vi "ProfilerTest.vi"() -> ()   [LabVIEW 2014] (continued)
{"Time"=28.20000000000161, "delVelocity"=0.0}, {"Time"=28.21000000000161, "delVelocity"=0.0}, {"Time"=28.220000000001612, "delVelocity"=0.0}, {"Time"=28.230000000001613, "delVelocity"=0.0}, {"Time"=28.240000000001615, "delVelocity"=0.0}, {"Time"=28.250000000001616, "delVelocity"=0.0}, {"Time"=28.260000000001618, "delVelocity"=0.0}, {"Time"=28.27000000000162, "delVelocity"=0.0}, {"Time"=28.28000000000162, "delVelocity"=0.0}, {"Time"=28.290000000001623, "delVelocity"=0.0}, {"Time"=28.300000000001624, "delVelocity"=0.0}, {"Time"=28.310000000001626, "delVelocity"=0.0}, {"Time"=28.320000000001627, "delVelocity"=0.0}, {"Time"=28.33000000000163, "delVelocity"=0.0}, {"Time"=28.34000000000163, "delVelocity"=0.0}, {"Time"=28.350000000001632, "delVelocity"=0.0}, {"Time"=28.360000000001634, "delVelocity"=0.0}, {"Time"=28.370000000001635, "delVelocity"=0.0}, {"Time"=28.380000000001637, "delVelocity"=0.0}, {"Time"=28.39000000000164, "delVelocity"=0.0}, {"Time"=28.40000000000164, "delVelocity"=0.0}, {"Time"=28.41000000000164, "delVelocity"=0.0}, {"Time"=28.420000000001643, "delVelocity"=0.0}, {"Time"=28.430000000001645, "delVelocity"=0.0}, {"Time"=28.440000000001646, "delVelocity"=0.0}, {"Time"=28.450000000001648, "delVelocity"=0.0}, {"Time"=28.46000000000165, "delVelocity"=0.0}, {"Time"=28.47000000000165, "delVelocity"=0.0}, {"Time"=28.480000000001652, "delVelocity"=0.0}, {"Time"=28.490000000001654, "delVelocity"=0.0}, {"Time"=28.500000000001656, "delVelocity"=0.0}, {"Time"=28.510000000001657, "delVelocity"=0.0}, {"Time"=28.52000000000166, "delVelocity"=0.0}, {"Time"=28.53000000000166, "delVelocity"=0.0}, {"Time"=28.540000000001662, "delVelocity"=0.0}, {"Time"=28.550000000001663, "delVelocity"=0.0}, {"Time"=28.560000000001665, "delVelocity"=0.0}, {"Time"=28.570000000001667, "delVelocity"=0.0}, {"Time"=28.580000000001668, "delVelocity"=0.0}, {"Time"=28.59000000000167, "delVelocity"=0.0}, {"Time"=28.60000000000167, "delVelocity"=0.0}, {"Time"=28.610000000001673, "delVelocity"=0.0}, {"Time"=28.620000000001674, "delVelocity"=0.0}, {"Time"=28.630000000001676, "delVelocity"=0.0}, {"Time"=28.640000000001677, "delVelocity"=0.0}, {"Time"=28.65000000000168, "delVelocity"=0.0}, {"Time"=28.66000000000168, "delVelocity"=0.0}, {"Time"=28.670000000001682, "delVelocity"=0.0}, {"Time"=28.680000000001684, "delVelocity"=0.0}, {"Time"=28.690000000001685, "delVelocity"=0.0}, {"Time"=28.700000000001687, "delVelocity"=0.0}, {"Time"=28.71000000000169, "delVelocity"=0.0}, {"Time"=28.72000000000169, "delVelocity"=0.0}, {"Time"=28.73000000000169, "delVelocity"=0.0}, {"Time"=28.740000000001693, "delVelocity"=0.0}, {"Time"=28.750000000001695, "delVelocity"=0.0}, {"Time"=28.760000000001696, "delVelocity"=0.0}, {"Time"=28.770000000001698, "delVelocity"=0.0}, {"Time"=28.7800000000017, "delVelocity"=0.0}, {"Time"=28.7900000000017, "delVelocity"=0.0}, {"Time"=28.800000000001702, "delVelocity"=0.0}, {"Time"=28.810000000001704, "delVelocity"=0.0}, {"Time"=28.820000000001706, "delVelocity"=0.0}, {"Time"=28.830000000001707, "delVelocity"=0.0}, {"Time"=28.84000000000171, "delVelocity"=0.0}, {"Time"=28.85000000000171, "delVelocity"=0.0}, {"Time"=28.860000000001712, "delVelocity"=0.0}, {"Time"=28.870000000001713, "delVelocity"=0.0}, {"Time"=28.880000000001715, "delVelocity"=0.0}, {"Time"=28.890000000001717, "delVelocity"=0.0}, {"Time"=28.900000000001718, "delVelocity"=0.0}, {"Time"=28.91000000000172, "delVelocity"=0.0}, {"Time"=28.92000000000172, "delVelocity"=0.0}, {"Time"=28.930000000001723, "delVelocity"=0.0}, {"Time"=28.940000000001724, "delVelocity"=0.0}, {"Time"=28.950000000001726, "delVelocity"=0.0}, {"Time"=28.960000000001727, "delVelocity"=0.0}, {"Time"=28.97000000000173, "delVelocity"=0.0}, {"Time"=28.98000000000173, "delVelocity"=0.0}, {"Time"=28.990000000001732, "delVelocity"=0.0}, {"Time"=29.000000000001734, "delVelocity"=0.0}, {"Time"=29.010000000001735, "delVelocity"=0.0}, {"Time"=29.020000000001737, "delVelocity"=0.0}, {"Time"=29.03000000000174, "delVelocity"=0.0}, {"Time"=29.04000000000174, "delVelocity"=0.0}, {"Time"=29.05000000000174, "delVelocity"=0.0}, {"Time"=29.060000000001743, "delVelocity"=0.0}, {"Time"=29.070000000001745, "delVelocity"=0.0}, {"Time"=29.080000000001746, "delVelocity"=0.0}, {"Time"=29.090000000001748, "delVelocity"=0.0}, {"Time"=29.10000000000175, "delVelocity"=0.0}, {"Time"=29.11000000000175, "delVelocity"=0.0}, {"Time"=29.120000000001752, "delVelocity"=0.0}, {"Time"=29.130000000001754, "delVelocity"=0.0}, {"Time"=29.140000000001756, "delVelocity"=0.0}, {"Time"=29.150000000001757, "delVelocity"=0.0}, {"Time"=29.16000000000176, "delVelocity"=0.0}, {"Time"=29.17000000000176, "delVelocity"=0.0}, {"Time"=29.180000000001762, "delVelocity"=0.0}, {"Time"=29.190000000001763, "delVelocity"=0.0}, {"Time"=29.200000000001765, "delVelocity"=0.0}, {"Time"=29.210000000001767, "delVelocity"=0.0}, {"Time"=29.220000000001768, "delVelocity"=0.0}, {"Time"=29.23000000000177, "delVelocity"=0.0}, {"Time"=29.24000000000177, "delVelocity"=0.0}, {"Time"=29.250000000001773, "delVelocity"=0.0}, {"Time"=29.260000000001774, "delVelocity"=0.0}, {"Time"=29.270000000001776, "delVelocity"=0.0}, {"Time"=29.280000000001777, "delVelocity"=0.0}, {"Time"=29.29000000000178, "delVelocity"=0.0}, {"Time"=29.30000000000178, "delVelocity"=0.0}, {"Time"=29.310000000001782, "delVelocity"=0.0}, {"Time"=29.320000000001784, "delVelocity"=0.0}, {"Time"=29.330000000001785, "delVelocity"=0.0}, {"Time"=29.340000000001787, "delVelocity"=0.0}, {"Time"=29.35000000000179, "delVelocity"=0.0}, {"Time"=29.36000000000179, "delVelocity"=0.0}, {"Time"=29.37000000000179, "delVelocity"=0.0}, {"Time"=29.380000000001793, "delVelocity"=0.0}, {"Time"=29.390000000001795, "delVelocity"=0.0}, {"Time"=29.400000000001796, "delVelocity"=0.0}, {"Time"=29.410000000001798, "delVelocity"=0.0}, {"Time"=29.4200000000018, "delVelocity"=0.0}, {"Time"=29.4300000000018, "delVelocity"=0.0}, {"Time"=29.440000000001803, "delVelocity"=0.0}, {"Time"=29.450000000001804, "delVelocity"=0.0}, {"Time"=29.460000000001806, "delVelocity"=0.0}, {"Time"=29.470000000001807, "delVelocity"=0.0}, {"Time"=29.48000000000181, "delVelocity"=0.0}, {"Time"=29.49000000000181, "delVelocity"=0.0}, {"Time"=29.500000000001812, "delVelocity"=0.0}, {"Time"=29.510000000001813, "delVelocity"=0.0}, {"Time"=29.520000000001815, "delVelocity"=0.0}, {"Time"=29.530000000001817, "delVelocity"=0.0}, {"Time"=29.540000000001818, "delVelocity"=0.0}, {"Time"=29.55000000000182, "delVelocity"=0.0}, {"Time"=29.56000000000182, "delVelocity"=0.0}, {"Time"=29.570000000001823, "delVelocity"=0.0}, {"Time"=29.580000000001824, "delVelocity"=0.0}, {"Time"=29.590000000001826, "delVelocity"=0.0}, {"Time"=29.600000000001828, "delVelocity"=0.0}, {"Time"=29.61000000000183, "delVelocity"=0.0}, {"Time"=29.62000000000183, "delVelocity"=0.0}, {"Time"=29.630000000001832, "delVelocity"=0.0}, {"Time"=29.640000000001834, "delVelocity"=0.0}, {"Time"=29.650000000001835, "delVelocity"=0.0}, {"Time"=29.660000000001837, "delVelocity"=0.0}, {"Time"=29.67000000000184, "delVelocity"=0.0}, {"Time"=29.68000000000184, "delVelocity"=0.0}, {"Time"=29.69000000000184, "delVelocity"=0.0}, {"Time"=29.700000000001843, "delVelocity"=0.0}, {"Time"=29.710000000001845, "delVelocity"=0.0}, {"Time"=29.720000000001846, "delVelocity"=0.0}, {"Time"=29.730000000001848, "delVelocity"=0.0}, {"Time"=29.74000000000185, "delVelocity"=0.0}, {"Time"=29.75000000000185, "delVelocity"=0.0}, {"Time"=29.760000000001853, "delVelocity"=0.0}, {"Time"=29.770000000001854, "delVelocity"=0.0}, {"Time"=29.780000000001856, "delVelocity"=0.0}, {"Time"=29.790000000001857, "delVelocity"=0.0}, {"Time"=29.80000000000186, "delVelocity"=0.0}, {"Time"=29.81000000000186, "delVelocity"=0.0}, {"Time"=29.820000000001862, "delVelocity"=0.0}, {"Time"=29.830000000001863, "delVelocity"=0.0}, {"Time"=29.840000000001865, "delVelocity"=0.0}, {"Time"=29.850000000001867, "delVelocity"=0.0}, {"Time"=29.860000000001868, "delVelocity"=0.0}, {"Time"=29.87000000000187, "delVelocity"=0.0}, {"Time"=29.88000000000187, "delVelocity"=0.0}, {"Time"=29.890000000001873, "delVelocity"=0.0}, {"Time"=29.900000000001874, "delVelocity"=0.0}, {"Time"=29.910000000001876, "delVelocity"=0.0}, {"Time"=29.920000000001878, "delVelocity"=0.0}, {"Time"=29.93000000000188, "delVelocity"=0.0}, {"Time"=29.94000000000188, "delVelocity"=0.0}, {"Time"=29.950000000001882, "delVelocity"=0.0}, {"Time"=29.960000000001884, "delVelocity"=0.0}, {"Time"=29.970000000001885, "delVelocity"=0.0}, {"Time"=29.980000000001887, "delVelocity"=0.0}, {"Time"=29.99000000000189, "delVelocity"=0.0}, {"Time"=30.00000000000189, "delVelocity"=0.0}, {"Time"=30.01000000000189, "delVelocity"=0.0}, {"Time"=30.020000000001893, "delVelocity"=0.0}, {"Time"=30.030000000001895, "delVelocity"=0.0}, {"Time"=30.040000000001896, "delVelocity"=0.0}, {"Time"=30.050000000001898, "delVelocity"=0.0}, {"Time"=30.0600000000019, "delVelocity"=0.0}, {"Time"=30.0700000000019, "delVelocity"=0.0}, {"Time"=30.080000000001903, "delVelocity"=0.0}, {"Time"=30.090000000001904, "delVelocity"=0.0}, {"Time"=30.100000000001906, "delVelocity"=0.0}, {"Time"=30.110000000001907, "delVelocity"=0.0}, {"Time"=30.12000000000191, "delVelocity"=0.0}, {"Time"=30.13000000000191, "delVelocity"=0.0}, {"Time"=30.140000000001912, "delVelocity"=0.0}, {"Time"=30.150000000001913, "delVelocity"=0.0}, {"Time"=30.160000000001915, "delVelocity"=0.0}, {"Time"=30.170000000001917, "delVelocity"=0.0}, {"Time"=30.180000000001918, "delVelocity"=0.0}, {"Time"=30.19000000000192, "delVelocity"=0.0}, {"Time"=30.20000000000192, "delVelocity"=0.0}, {"Time"=30.210000000001923, "delVelocity"=0.0}, {"Time"=30.220000000001924, "delVelocity"=0.0}, {"Time"=30.230000000001926, "delVelocity"=0.0}, {"Time"=30.240000000001928, "delVelocity"=0.0}, {"Time"=30.25000000000193, "delVelocity"=0.0}, {"Time"=30.26000000000193, "delVelocity"=0.0}, {"Time"=30.270000000001932, "delVelocity"=0.0}, {"Time"=30.280000000001934, "delVelocity"=0.0}, {"Time"=30.290000000001935, "delVelocity"=0.0}, {"Time"=30.300000000001937, "delVelocity"=0.0}, {"Time"=30.31000000000194, "delVelocity"=0.0}, {"Time"=30.32000000000194, "delVelocity"=0.0}, {"Time"=30.33000000000194, "delVelocity"=0.0}, {"Time"=30.340000000001943, "delVelocity"=0.0}, {"Time"=30.350000000001945, "delVelocity"=0.0}, {"Time"=30.360000000001946, "delVelocity"=0.0}, {"Time"=30.370000000001948, "delVelocity"=0.0}, {"Time"=30.38000000000195, "delVelocity"=0.0}, {"Time"=30.39000000000195, "delVelocity"=0.0}, {"Time"=30.400000000001953, "delVelocity"=0.0}, {"Time"=30.410000000001954, "delVelocity"=0.0}, {"Time"=30.420000000001956, "delVelocity"=0.0}, {"Time"=30.430000000001957, "delVelocity"=0.0}, {"Time"=30.44000000000196, "delVelocity"=0.0}, {"Time"=30.45000000000196, "delVelocity"=0.0}, {"Time"=30.460000000001962, "delVelocity"=0.0}, {"Time"=30.470000000001964, "delVelocity"=0.0}, {"Time"=30.480000000001965, "delVelocity"=0.0}, {"Time"=30.490000000001967, "delVelocity"=0.0}, {"Time"=30.500000000001968, "delVelocity"=0.0}, {"Time"=30.51000000000197, "delVelocity"=0.0}, {"Time"=30.52000000000197, "delVelocity"=0.0}, {"Time"=30.530000000001973, "delVelocity"=0.0}, {"Time"=30.540000000001974, "delVelocity"=0.0}, {"Time"=30.550000000001976, "delVelocity"=0.0}, {"Time"=30.560000000001978, "delVelocity"=0.0}, {"Time"=30.57000000000198, "delVelocity"=0.0}, {"Time"=30.58000000000198, "delVelocity"=0.0}, {"Time"=30.590000000001982, "delVelocity"=0.0}, {"Time"=30.600000000001984, "delVelocity"=0.0}, {"Time"=30.610000000001985, "delVelocity"=0.0}, {"Time"=30.620000000001987, "delVelocity"=0.0}, {"Time"=30.63000000000199, "delVelocity"=0.0}, {"Time"=30.64000000000199, "delVelocity"=0.0}, {"Time"=30.65000000000199, "delVelocity"=0.0}, {"Time"=30.660000000001993, "delVelocity"=0.0}, {"Time"=30.670000000001995, "delVelocity"=0.0}, {"Time"=30.680000000001996, "delVelocity"=0.0}, {"Time"=30.690000000001998, "delVelocity"=0.0}, {"Time"=30.700000000002, "delVelocity"=0.0}, {"Time"=30.710000000002, "delVelocity"=0.0}, {"Time"=30.720000000002003, "delVelocity"=0.0}, {"Time"=30.730000000002004, "delVelocity"=0.0}, {"Time"=30.740000000002006, "delVelocity"=0.0}, {"Time"=30.750000000002007, "delVelocity"=0.0}, {"Time"=30.76000000000201, "delVelocity"=0.0}, {"Time"=30.77000000000201, "delVelocity"=0.0}, {"Time"=30.780000000002012, "delVelocity"=0.0}, {"Time"=30.790000000002014, "delVelocity"=0.0}, {"Time"=30.800000000002015, "delVelocity"=0.0}, {"Time"=30.810000000002017, "delVelocity"=0.0}, {"Time"=30.82000000000202, "delVelocity"=0.0}, {"Time"=30.83000000000202, "delVelocity"=0.0}, {"Time"=30.84000000000202, "delVelocity"=0.0}, {"Time"=30.850000000002023, "delVelocity"=0.0}, {"Time"=30.860000000002024, "delVelocity"=0.0}, {"Time"=30.870000000002026, "delVelocity"=0.0}, {"Time"=30.880000000002028, "delVelocity"=0.0}, {"Time"=30.89000000000203, "delVelocity"=0.0}, {"Time"=30.90000000000203, "delVelocity"=0.0}, {"Time"=30.910000000002032, "delVelocity"=0.0}, {"Time"=30.920000000002034, "delVelocity"=0.0}, {"Time"=30.930000000002035, "delVelocity"=0.0}, {"Time"=30.940000000002037, "delVelocity"=0.0}, {"Time"=30.95000000000204, "delVelocity"=0.0}, {"Time"=30.96000000000204, "delVelocity"=0.0}, {"Time"=30.97000000000204, "delVelocity"=0.0}, {"Time"=30.980000000002043, "delVelocity"=0.0}, {"Time"=30.990000000002045, "delVelocity"=0.0}, {"Time"=31.000000000002046, "delVelocity"=0.0}, {"Time"=31.010000000002048, "delVelocity"=0.0}, {"Time"=31.02000000000205, "delVelocity"=0.0}, {"Time"=31.03000000000205, "delVelocity"=0.0}, {"Time"=31.040000000002053, "delVelocity"=0.0}, {"Time"=31.050000000002054, "delVelocity"=0.0}, {"Time"=31.060000000002056, "delVelocity"=0.0}, {"Time"=31.070000000002057, "delVelocity"=0.0}, {"Time"=31.08000000000206, "delVelocity"=0.0}, {"Time"=31.09000000000206, "delVelocity"=0.0}, {"Time"=31.100000000002062, "delVelocity"=0.0}, {"Time"=31.110000000002064, "delVelocity"=0.0}, {"Time"=31.120000000002065, "delVelocity"=0.0}, {"Time"=31.130000000002067, "delVelocity"=0.0}, {"Time"=31.14000000000207, "delVelocity"=0.0}, {"Time"=31.15000000000207, "delVelocity"=0.0}, {"Time"=31.16000000000207, "delVelocity"=0.0}, {"Time"=31.170000000002073, "delVelocity"=0.0}, {"Time"=31.180000000002075, "delVelocity"=0.0}, {"Time"=31.190000000002076, "delVelocity"=0.0}, {"Time"=31.200000000002078, "delVelocity"=0.0}, {"Time"=31.21000000000208, "delVelocity"=0.0}, {"Time"=31.22000000000208, "delVelocity"=0.0}, {"Time"=31.230000000002082, "delVelocity"=0.0}, {"Time"=31.240000000002084, "delVelocity"=0.0}, {"Time"=31.250000000002085, "delVelocity"=0.0}, {"Time"=31.260000000002087, "delVelocity"=0.0}, {"Time"=31.27000000000209, "delVelocity"=0.0}, {"Time"=31.28000000000209, "delVelocity"=0.0}, {"Time"=31.29000000000209, "delVelocity"=0.0}, {"Time"=31.300000000002093, "delVelocity"=0.0}, {"Time"=31.310000000002095, "delVelocity"=0.0}, {"Time"=31.320000000002096, "delVelocity"=0.0}, {"Time"=31.330000000002098, "delVelocity"=0.0}, {"Time"=31.3400000000021, "delVelocity"=0.0}, {"Time"=31.3500000000021, "delVelocity"=0.0}, {"Time"=31.360000000002103, "delVelocity"=0.0}, {"Time"=31.370000000002104, "delVelocity"=0.0}, {"Time"=31.380000000002106, "delVelocity"=0.0}, {"Time"=31.390000000002107, "delVelocity"=0.0}, {"Time"=31.40000000000211, "delVelocity"=0.0}, {"Time"=31.41000000000211, "delVelocity"=0.0}, {"Time"=31.420000000002112, "delVelocity"=0.0}, {"Time"=31.430000000002114, "delVelocity"=0.0}, {"Time"=31.440000000002115, "delVelocity"=0.0}, {"Time"=31.450000000002117, "delVelocity"=0.0}, {"Time"=31.46000000000212, "delVelocity"=0.0}, {"Time"=31.47000000000212, "delVelocity"=0.0}, {"Time"=31.48000000000212, "delVelocity"=0.0}, {"Time"=31.490000000002123, "delVelocity"=0.0}, {"Time"=31.500000000002125, "delVelocity"=0.0}, {"Time"=31.510000000002126, "delVelocity"=0.0}, {"Time"=31.520000000002128, "delVelocity"=0.0}, {"Time"=31.53000000000213, "delVelocity"=0.0}, {"Time"=31.54000000000213, "delVelocity"=0.0}, {"Time"=31.550000000002132, "delVelocity"=0.0}, {"Time"=31.560000000002134, "delVelocity"=0.0}, {"Time"=31.570000000002135, "delVelocity"=0.0}, {"Time"=31.580000000002137, "delVelocity"=0.0}, {"Time"=31.59000000000214, "delVelocity"=0.0}, {"Time"=31.60000000000214, "delVelocity"=0.0}, {"Time"=31.61000000000214, "delVelocity"=0.0}, {"Time"=31.620000000002143, "delVelocity"=0.0}, {"Time"=31.630000000002145, "delVelocity"=0.0}, {"Time"=31.640000000002146, "delVelocity"=0.0}, {"Time"=31.650000000002148, "delVelocity"=0.0}, {"Time"=31.66000000000215, "delVelocity"=0.0}, {"Time"=31.67000000000215, "delVelocity"=0.0}, {"Time"=31.680000000002153, "delVelocity"=0.0}, {"Time"=31.690000000002154, "delVelocity"=0.0}, {"Time"=31.700000000002156, "delVelocity"=0.0}, {"Time"=31.710000000002157, "delVelocity"=0.0}, {"Time"=31.72000000000216, "delVelocity"=0.0}, {"Time"=31.73000000000216, "delVelocity"=0.0}, {"Time"=31.740000000002162, "delVelocity"=0.0}, {"Time"=31.750000000002164, "delVelocity"=0.0}, {"Time"=31.760000000002165, "delVelocity"=0.0}, {"Time"=31.770000000002167, "delVelocity"=0.0}, {"Time"=31.78000000000217, "delVelocity"=0.0}, {"Time"=31.79000000000217, "delVelocity"=0.0}, {"Time"=31.80000000000217, "delVelocity"=0.0}, {"Time"=31.810000000002173, "delVelocity"=0.0}, {"Time"=31.820000000002175, "delVelocity"=0.0}, {"Time"=31.830000000002176, "delVelocity"=0.0}, {"Time"=31.840000000002178, "delVelocity"=0.0}, {"Time"=31.85000000000218, "delVelocity"=0.0}, {"Time"=31.86000000000218, "delVelocity"=0.0}, {"Time"=31.870000000002182, "delVelocity"=0.0}, {"Time"=31.880000000002184, "delVelocity"=0.0}, {"Time"=31.890000000002185, "delVelocity"=0.0}, {"Time"=31.900000000002187, "delVelocity"=0.0}, {"Time"=31.91000000000219, "delVelocity"=0.0}, {"Time"=31.92000000000219, "delVelocity"=0.0}, {"Time"=31.93000000000219, "delVelocity"=0.0}, {"Time"=31.940000000002193, "delVelocity"=0.0}, {"Time"=31.950000000002195, "delVelocity"=0.0}, {"Time"=31.960000000002196, "delVelocity"=0.0}, {"Time"=31.970000000002198, "delVelocity"=0.0}, {"Time"=31.9800000000022, "delVelocity"=0.0}, {"Time"=31.9900000000022, "delVelocity"=0.0}, {"Time"=32.0000000000022, "delVelocity"=0.0}, {"Time"=32.0100000000022, "delVelocity"=0.0}, {"Time"=32.0200000000022, "delVelocity"=0.0}, {"Time"=32.0300000000022, "delVelocity"=0.0}, {"Time"=32.040000000002195, "delVelocity"=0.0}, {"Time"=32.05000000000219, "delVelocity"=0.0}, {"Time"=32.06000000000219, "delVelocity"=0.0}, {"Time"=32.07000000000219, "delVelocity"=0.0}, {"Time"=32.08000000000219, "delVelocity"=0.0}, {"Time"=32.090000000002185, "delVelocity"=0.0}, {"Time"=32.10000000000218, "delVelocity"=0.0}, {"Time"=32.11000000000218, "delVelocity"=0.0}, {"Time"=32.12000000000218, "delVelocity"=0.0}, {"Time"=32.13000000000218, "delVelocity"=0.0}, {"Time"=32.140000000002175, "delVelocity"=0.0}, {"Time"=32.15000000000217, "delVelocity"=0.0}, {"Time"=32.16000000000217, "delVelocity"=0.0}, {"Time"=32.17000000000217, "delVelocity"=0.0}, {"Time"=32.18000000000217, "delVelocity"=0.0}, {"Time"=32.190000000002165, "delVelocity"=0.0}, {"Time"=32.20000000000216, "delVelocity"=0.0}, {"Time"=32.21000000000216, "delVelocity"=0.0}, {"Time"=32.22000000000216, "delVelocity"=0.0}, {"Time"=32.23000000000216, "delVelocity"=0.0}, {"Time"=32.240000000002155, "delVelocity"=0.0}, {"Time"=32.25000000000215, "delVelocity"=0.0}, {"Time"=32.26000000000215, "delVelocity"=0.0}, {"Time"=32.27000000000215, "delVelocity"=0.0}, {"Time"=32.28000000000215, "delVelocity"=0.0}, {"Time"=32.290000000002145, "delVelocity"=0.0}, {"Time"=32.30000000000214, "delVelocity"=0.0}, {"Time"=32.31000000000214, "delVelocity"=0.0}, {"Time"=32.32000000000214, "delVelocity"=0.0}, {"Time"=32.33000000000214, "delVelocity"=0.0}, {"Time"=32.340000000002135, "delVelocity"=0.0}, {"Time"=32.35000000000213, "delVelocity"=0.0}, {"Time"=32.36000000000213, "delVelocity"=0.0}, {"Time"=32.37000000000213, "delVelocity"=0.0}, {"Time"=32.38000000000213, "delVelocity"=0.0}, {"Time"=32.390000000002125, "delVelocity"=0.0}, {"Time"=32.40000000000212, "delVelocity"=0.0}, {"Time"=32.41000000000212, "delVelocity"=0.0}, {"Time"=32.42000000000212, "delVelocity"=0.0}, {"Time"=32.43000000000212, "delVelocity"=0.0}, {"Time"=32.440000000002115, "delVelocity"=0.0}, {"Time"=32.45000000000211, "delVelocity"=0.0}, {"Time"=32.46000000000211, "delVelocity"=0.0}, {"Time"=32.47000000000211, "delVelocity"=0.0}, {"Time"=32.48000000000211, "delVelocity"=0.0}, {"Time"=32.490000000002105, "delVelocity"=0.0}, {"Time"=32.5000000000021, "delVelocity"=0.0}, {"Time"=32.5100000000021, "delVelocity"=0.0}, {"Time"=32.5200000000021, "delVelocity"=0.0}, {"Time"=32.5300000000021, "delVelocity"=0.0}, {"Time"=32.540000000002095, "delVelocity"=0.0}, {"Time"=32.55000000000209, "delVelocity"=0.0}, {"Time"=32.56000000000209, "delVelocity"=0.0}, {"Time"=32.57000000000209, "delVelocity"=0.0}, {"Time"=32.58000000000209, "delVelocity"=0.0}, {"Time"=32.590000000002085, "delVelocity"=0.0}, {"Time"=32.60000000000208, "delVelocity"=0.0}, {"Time"=32.61000000000208, "delVelocity"=0.0}, {"Time"=32.62000000000208, "delVelocity"=0.0}, {"Time"=32.63000000000208, "delVelocity"=0.0}, {"Time"=32.640000000002075, "delVelocity"=0.0}, {"Time"=32.65000000000207, "delVelocity"=0.0}, {"Time"=32.66000000000207, "delVelocity"=0.0}, {"Time"=32.67000000000207, "delVelocity"=0.0}, {"Time"=32.68000000000207, "delVelocity"=0.0}, {"Time"=32.690000000002065, "delVelocity"=0.0}, {"Time"=32.70000000000206, "delVelocity"=0.0}, {"Time"=32.71000000000206, "delVelocity"=0.0}, {"Time"=32.72000000000206, "delVelocity"=0.0}, {"Time"=32.73000000000206, "delVelocity"=0.0}, {"Time"=32.740000000002055, "delVelocity"=0.0}, {"Time"=32.75000000000205, "delVelocity"=0.0}, {"Time"=32.76000000000205, "delVelocity"=0.0}, {"Time"=32.77000000000205, "delVelocity"=0.0}, {"Time"=32.78000000000205, "delVelocity"=0.0}, {"Time"=32.790000000002046, "delVelocity"=0.0}, {"Time"=32.80000000000204, "delVelocity"=0.0}, {"Time"=32.81000000000204, "delVelocity"=0.0}, {"Time"=32.82000000000204, "delVelocity"=0.0}, {"Time"=32.83000000000204, "delVelocity"=0.0}, {"Time"=32.840000000002036, "delVelocity"=0.0}, {"Time"=32.850000000002034, "delVelocity"=0.0}, {"Time"=32.86000000000203, "delVelocity"=0.0}, {"Time"=32.87000000000203, "delVelocity"=0.0}, {"Time"=32.88000000000203, "delVelocity"=0.0}, {"Time"=32.890000000002026, "delVelocity"=0.0}, {"Time"=32.900000000002024, "delVelocity"=0.0}, {"Time"=32.91000000000202, "delVelocity"=0.0}, {"Time"=32.92000000000202, "delVelocity"=0.0}, {"Time"=32.93000000000202, "delVelocity"=0.0}, {"Time"=32.940000000002016, "delVelocity"=0.0}, {"Time"=32.950000000002014, "delVelocity"=0.0}, {"Time"=32.96000000000201, "delVelocity"=0.0}, {"Time"=32.97000000000201, "delVelocity"=0.0}, {"Time"=32.98000000000201, "delVelocity"=0.0}, {"Time"=32.990000000002006, "delVelocity"=0.0}, {"Time"=33.000000000002004, "delVelocity"=0.0}, {"Time"=33.010000000002, "delVelocity"=0.0}, {"Time"=33.020000000002, "delVelocity"=0.0}, {"Time"=33.030000000002, "delVelocity"=0.0}, {"Time"=33.040000000001996, "delVelocity"=0.0}, {"Time"=33.050000000001994, "delVelocity"=0.0}, {"Time"=33.06000000000199, "delVelocity"=0.0}, {"Time"=33.07000000000199, "delVelocity"=0.0}, {"Time"=33.08000000000199, "delVelocity"=0.0}, {"Time"=33.090000000001986, "delVelocity"=0.0}, {"Time"=33.100000000001984, "delVelocity"=0.0}, {"Time"=33.11000000000198, "delVelocity"=0.0}, {"Time"=33.12000000000198, "delVelocity"=0.0}, {"Time"=33.13000000000198, "delVelocity"=0.0}, {"Time"=33.140000000001976, "delVelocity"=0.0}, {"Time"=33.150000000001974, "delVelocity"=0.0}, {"Time"=33.16000000000197, "delVelocity"=0.0}, {"Time"=33.17000000000197, "delVelocity"=0.0}, {"Time"=33.18000000000197, "delVelocity"=0.0}, {"Time"=33.190000000001966, "delVelocity"=0.0}, {"Time"=33.200000000001964, "delVelocity"=0.0}, {"Time"=33.21000000000196, "delVelocity"=0.0}, {"Time"=33.22000000000196, "delVelocity"=0.0}, {"Time"=33.23000000000196, "delVelocity"=0.0}, {"Time"=33.240000000001956, "delVelocity"=0.0}, {"Time"=33.250000000001954, "delVelocity"=0.0}, {"Time"=33.26000000000195, "delVelocity"=0.0}, {"Time"=33.27000000000195, "delVelocity"=0.0}, {"Time"=33.28000000000195, "delVelocity"=0.0}, {"Time"=33.290000000001946, "delVelocity"=0.0}, {"Time"=33.300000000001944, "delVelocity"=0.0}, {"Time"=33.31000000000194, "delVelocity"=0.0}, {"Time"=33.32000000000194, "delVelocity"=0.0}, {"Time"=33.33000000000194, "delVelocity"=0.0}, {"Time"=33.340000000001936, "delVelocity"=0.0}, {"Time"=33.350000000001934, "delVelocity"=0.0}, {"Time"=33.36000000000193, "delVelocity"=0.0}, {"Time"=33.37000000000193, "delVelocity"=0.0}, {"Time"=33.38000000000193, "delVelocity"=0.0}, {"Time"=33.390000000001926, "delVelocity"=0.0}, {"Time"=33.400000000001924, "delVelocity"=0.0}, {"Time"=33.41000000000192, "delVelocity"=0.0}, {"Time"=33.42000000000192, "delVelocity"=0.0}, {"Time"=33.43000000000192, "delVelocity"=0.0}, {"Time"=33.440000000001916, "delVelocity"=0.0}, {"Time"=33.450000000001914, "delVelocity"=0.0}, {"Time"=33.46000000000191, "delVelocity"=0.0}, {"Time"=33.47000000000191, "delVelocity"=0.0}, {"Time"=33.48000000000191, "delVelocity"=0.0}, {"Time"=33.490000000001906, "delVelocity"=0.0}, {"Time"=33.500000000001904, "delVelocity"=0.0}, {"Time"=33.5100000000019, "delVelocity"=0.0}, {"Time"=33.5200000000019, "delVelocity"=0.0}, {"Time"=33.5300000000019, "delVelocity"=0.0}, {"Time"=33.540000000001896, "delVelocity"=0.0}, {"Time"=33.550000000001894, "delVelocity"=0.0}, {"Time"=33.56000000000189, "delVelocity"=0.0}, {"Time"=33.57000000000189, "delVelocity"=0.0}, {"Time"=33.58000000000189, "delVelocity"=0.0}, {"Time"=33.590000000001886, "delVelocity"=0.0}, {"Time"=33.600000000001884, "delVelocity"=0.0}, {"Time"=33.61000000000188, "delVelocity"=0.0}, {"Time"=33.62000000000188, "delVelocity"=0.0}, {"Time"=33.63000000000188, "delVelocity"=0.0}, {"Time"=33.640000000001876, "delVelocity"=0.0}, {"Time"=33.650000000001874, "delVelocity"=0.0}, {"Time"=33.66000000000187, "delVelocity"=0.0}, {"Time"=33.67000000000187, "delVelocity"=0.0}, {"Time"=33.68000000000187, "delVelocity"=0.0}, {"Time"=33.69000000000187, "delVelocity"=0.0}, {"Time"=33.700000000001864, "delVelocity"=0.0}, {"Time"=33.71000000000186, "delVelocity"=0.0}, {"Time"=33.72000000000186, "delVelocity"=0.0}, {"Time"=33.73000000000186, "delVelocity"=0.0}, {"Time"=33.74000000000186, "delVelocity"=0.0}, {"Time"=33.750000000001855, "delVelocity"=0.0}, {"Time"=33.76000000000185, "delVelocity"=0.0}, {"Time"=33.77000000000185, "delVelocity"=0.0}, {"Time"=33.78000000000185, "delVelocity"=0.0}, {"Time"=33.79000000000185, "delVelocity"=0.0}, {"Time"=33.800000000001845, "delVelocity"=0.0}, {"Time"=33.81000000000184, "delVelocity"=0.0}, {"Time"=33.82000000000184, "delVelocity"=0.0}, {"Time"=33.83000000000184, "delVelocity"=0.0}, {"Time"=33.84000000000184, "delVelocity"=0.0}, {"Time"=33.850000000001835, "delVelocity"=0.0}, {"Time"=33.86000000000183, "delVelocity"=0.0}, {"Time"=33.87000000000183, "delVelocity"=0.0}, {"Time"=33.88000000000183, "delVelocity"=0.0}, {"Time"=33.89000000000183, "delVelocity"=0.0}, {"Time"=33.900000000001825, "delVelocity"=0.0}, {"Time"=33.91000000000182, "delVelocity"=0.0}, {"Time"=33.92000000000182, "delVelocity"=0.0}, {"Time"=33.93000000000182, "delVelocity"=0.0}, {"Time"=33.94000000000182, "delVelocity"=0.0}, {"Time"=33.950000000001815, "delVelocity"=0.0}, {"Time"=33.96000000000181, "delVelocity"=0.0}, {"Time"=33.97000000000181, "delVelocity"=0.0}, {"Time"=33.98000000000181, "delVelocity"=0.0}, {"Time"=33.99000000000181, "delVelocity"=0.0}, {"Time"=34.000000000001805, "delVelocity"=0.0}, {"Time"=34.0100000000018, "delVelocity"=0.0}, {"Time"=34.0200000000018, "delVelocity"=0.0}, {"Time"=34.0300000000018, "delVelocity"=0.0}, {"Time"=34.0400000000018, "delVelocity"=0.0}, {"Time"=34.050000000001795, "delVelocity"=0.0}, {"Time"=34.06000000000179, "delVelocity"=0.0}, {"Time"=34.07000000000179, "delVelocity"=0.0}, {"Time"=34.08000000000179, "delVelocity"=0.0}, {"Time"=34.09000000000179, "delVelocity"=0.0}, {"Time"=34.100000000001785, "delVelocity"=0.0}, {"Time"=34.11000000000178, "delVelocity"=0.0}, {"Time"=34.12000000000178, "delVelocity"=0.0}, {"Time"=34.13000000000178, "delVelocity"=0.0}, {"Time"=34.14000000000178, "delVelocity"=0.0}, {"Time"=34.150000000001775, "delVelocity"=0.0}, {"Time"=34.16000000000177, "delVelocity"=0.0}, {"Time"=34.17000000000177, "delVelocity"=0.0}, {"Time"=34.18000000000177, "delVelocity"=0.0}, {"Time"=34.19000000000177, "delVelocity"=0.0}, {"Time"=34.200000000001765, "delVelocity"=0.0}, {"Time"=34.21000000000176, "delVelocity"=0.0}, {"Time"=34.22000000000176, "delVelocity"=0.0}, {"Time"=34.23000000000176, "delVelocity"=0.0}, {"Time"=34.24000000000176, "delVelocity"=0.0}, {"Time"=34.250000000001755, "delVelocity"=0.0}, {"Time"=34.26000000000175, "delVelocity"=0.0}, {"Time"=34.27000000000175, "delVelocity"=0.0}, {"Time"=34.28000000000175, "delVelocity"=0.0}, {"Time"=34.29000000000175, "delVelocity"=0.0}, {"Time"=34.300000000001745, "delVelocity"=0.0}, {"Time"=34.31000000000174, "delVelocity"=0.0}, {"Time"=34.32000000000174, "delVelocity"=0.0}, {"Time"=34.33000000000174, "delVelocity"=0.0}, {"Time"=34.34000000000174, "delVelocity"=0.0}, {"Time"=34.350000000001735, "delVelocity"=0.0}, {"Time"=34.36000000000173, "delVelocity"=0.0}, {"Time"=34.37000000000173, "delVelocity"=0.0}, {"Time"=34.38000000000173, "delVelocity"=0.0}, {"Time"=34.39000000000173, "delVelocity"=0.0}, {"Time"=34.400000000001725, "delVelocity"=0.0}, {"Time"=34.41000000000172, "delVelocity"=0.0}, {"Time"=34.42000000000172, "delVelocity"=0.0}, {"Time"=34.43000000000172, "delVelocity"=0.0}, {"Time"=34.44000000000172, "delVelocity"=0.0}, {"Time"=34.450000000001715, "delVelocity"=0.0}, {"Time"=34.46000000000171, "delVelocity"=0.0}, {"Time"=34.47000000000171, "delVelocity"=0.0}, {"Time"=34.48000000000171, "delVelocity"=0.0}, {"Time"=34.49000000000171, "delVelocity"=0.0}, {"Time"=34.500000000001705, "delVelocity"=0.0}, {"Time"=34.5100000000017, "delVelocity"=0.0}, {"Time"=34.5200000000017, "delVelocity"=0.0}, {"Time"=34.5300000000017, "delVelocity"=0.0}, {"Time"=34.5400000000017, "delVelocity"=0.0}, {"Time"=34.550000000001695, "delVelocity"=0.0}, {"Time"=34.56000000000169, "delVelocity"=0.0}, {"Time"=34.57000000000169, "delVelocity"=0.0}, {"Time"=34.58000000000169, "delVelocity"=0.0}, {"Time"=34.59000000000169, "delVelocity"=0.0}, {"Time"=34.600000000001685, "delVelocity"=0.0}, {"Time"=34.61000000000168, "delVelocity"=0.0}, {"Time"=34.62000000000168, "delVelocity"=0.0}, {"Time"=34.63000000000168, "delVelocity"=0.0}, {"Time"=34.64000000000168, "delVelocity"=0.0}, {"Time"=34.650000000001675, "delVelocity"=0.0}, {"Time"=34.66000000000167, "delVelocity"=0.0}, {"Time"=34.67000000000167, "delVelocity"=0.0}, {"Time"=34.68000000000167, "delVelocity"=0.0}, {"Time"=34.69000000000167, "delVelocity"=0.0}, {"Time"=34.700000000001666, "delVelocity"=0.0}, {"Time"=34.71000000000166, "delVelocity"=0.0}, {"Time"=34.72000000000166, "delVelocity"=0.0}, {"Time"=34.73000000000166, "delVelocity"=0.0}, {"Time"=34.74000000000166, "delVelocity"=0.0}, {"Time"=34.750000000001656, "delVelocity"=0.0}, {"Time"=34.760000000001654, "delVelocity"=0.0}, {"Time"=34.77000000000165, "delVelocity"=0.0}, {"Time"=34.78000000000165, "delVelocity"=0.0}, {"Time"=34.79000000000165, "delVelocity"=0.0}, {"Time"=34.800000000001646, "delVelocity"=0.0}, {"Time"=34.810000000001644, "delVelocity"=0.0}, {"Time"=34.82000000000164, "delVelocity"=0.0}, {"Time"=34.83000000000164, "delVelocity"=0.0}, {"Time"=34.84000000000164, "delVelocity"=0.0}, {"Time"=34.850000000001636, "delVelocity"=0.0}, {"Time"=34.860000000001634, "delVelocity"=0.0}, {"Time"=34.87000000000163, "delVelocity"=0.0}, {"Time"=34.88000000000163, "delVelocity"=0.0}, {"Time"=34.89000000000163, "delVelocity"=0.0}, {"Time"=34.900000000001626, "delVelocity"=0.0}, {"Time"=34.910000000001624, "delVelocity"=0.0}, {"Time"=34.92000000000162, "delVelocity"=0.0}, {"Time"=34.93000000000162, "delVelocity"=0.0}, {"Time"=34.94000000000162, "delVelocity"=0.0}, {"Time"=34.950000000001616, "delVelocity"=0.0}, {"Time"=34.960000000001614, "delVelocity"=0.0}, {"Time"=34.97000000000161, "delVelocity"=0.0}, {"Time"=34.98000000000161, "delVelocity"=0.0}, {"Time"=34.99000000000161, "delVelocity"=0.0}, {"Time"=35.000000000001606, "delVelocity"=0.0}, {"Time"=35.010000000001604, "delVelocity"=0.0}, {"Time"=35.0200000000016, "delVelocity"=0.0}, {"Time"=35.0300000000016, "delVelocity"=0.0}, {"Time"=35.0400000000016, "delVelocity"=0.0}, {"Time"=35.050000000001596, "delVelocity"=0.0}, {"Time"=35.060000000001594, "delVelocity"=0.0}, {"Time"=35.07000000000159, "delVelocity"=0.0}, {"Time"=35.08000000000159, "delVelocity"=0.0}, {"Time"=35.09000000000159, "delVelocity"=0.0}, {"Time"=35.100000000001586, "delVelocity"=0.0}, {"Time"=35.110000000001584, "delVelocity"=0.0}, {"Time"=35.12000000000158, "delVelocity"=0.0}, {"Time"=35.13000000000158, "delVelocity"=0.0}, {"Time"=35.14000000000158, "delVelocity"=0.0}, {"Time"=35.150000000001576, "delVelocity"=0.0}, {"Time"=35.160000000001574, "delVelocity"=0.0}, {"Time"=35.17000000000157, "delVelocity"=0.0}, {"Time"=35.18000000000157, "delVelocity"=0.0}, {"Time"=35.19000000000157, "delVelocity"=0.0}, {"Time"=35.200000000001566, "delVelocity"=0.0}, {"Time"=35.210000000001564, "delVelocity"=0.0}, {"Time"=35.22000000000156, "delVelocity"=0.0}, {"Time"=35.23000000000156, "delVelocity"=0.0}, {"Time"=35.24000000000156, "delVelocity"=0.0}, {"Time"=35.250000000001556, "delVelocity"=0.0}, {"Time"=35.260000000001554, "delVelocity"=0.0}, {"Time"=35.27000000000155, "delVelocity"=0.0}, {"Time"=35.28000000000155, "delVelocity"=0.0}, {"Time"=35.29000000000155, "delVelocity"=0.0}, {"Time"=35.300000000001546, "delVelocity"=0.0}, {"Time"=35.310000000001544, "delVelocity"=0.0}, {"Time"=35.32000000000154, "delVelocity"=0.0}, {"Time"=35.33000000000154, "delVelocity"=0.0}, {"Time"=35.34000000000154, "delVelocity"=0.0}, {"Time"=35.350000000001536, "delVelocity"=0.0}, {"Time"=35.360000000001534, "delVelocity"=0.0}, {"Time"=35.37000000000153, "delVelocity"=0.0}, {"Time"=35.38000000000153, "delVelocity"=0.0}, {"Time"=35.39000000000153, "delVelocity"=0.0}, {"Time"=35.400000000001526, "delVelocity"=0.0}, {"Time"=35.410000000001524, "delVelocity"=0.0}, {"Time"=35.42000000000152, "delVelocity"=0.0}, {"Time"=35.43000000000152, "delVelocity"=0.0}, {"Time"=35.44000000000152, "delVelocity"=0.0}, {"Time"=35.450000000001516, "delVelocity"=0.0}, {"Time"=35.460000000001514, "delVelocity"=0.0}, {"Time"=35.47000000000151, "delVelocity"=0.0}, {"Time"=35.48000000000151, "delVelocity"=0.0}, {"Time"=35.49000000000151, "delVelocity"=0.0}, {"Time"=35.500000000001506, "delVelocity"=0.0}, {"Time"=35.510000000001504, "delVelocity"=0.0}, {"Time"=35.5200000000015, "delVelocity"=0.0}, {"Time"=35.5300000000015, "delVelocity"=0.0}, {"Time"=35.5400000000015, "delVelocity"=0.0}, {"Time"=35.550000000001496, "delVelocity"=0.0}, {"Time"=35.560000000001494, "delVelocity"=0.0}, {"Time"=35.57000000000149, "delVelocity"=0.0}, {"Time"=35.58000000000149, "delVelocity"=0.0}, {"Time"=35.59000000000149, "delVelocity"=0.0}, {"Time"=35.60000000000149, "delVelocity"=0.0}, {"Time"=35.610000000001484, "delVelocity"=0.0}, {"Time"=35.62000000000148, "delVelocity"=0.0}, {"Time"=35.63000000000148, "delVelocity"=0.0}, {"Time"=35.64000000000148, "delVelocity"=0.0}, {"Time"=35.65000000000148, "delVelocity"=0.0}, {"Time"=35.660000000001475, "delVelocity"=0.0}, {"Time"=35.67000000000147, "delVelocity"=0.0}, {"Time"=35.68000000000147, "delVelocity"=0.0}, {"Time"=35.69000000000147, "delVelocity"=0.0}, {"Time"=35.70000000000147, "delVelocity"=0.0}, {"Time"=35.710000000001465, "delVelocity"=0.0}, {"Time"=35.72000000000146, "delVelocity"=0.0}, {"Time"=35.73000000000146, "delVelocity"=0.0}, {"Time"=35.74000000000146, "delVelocity"=0.0}, {"Time"=35.75000000000146, "delVelocity"=0.0}, {"Time"=35.760000000001455, "delVelocity"=0.0}, {"Time"=35.77000000000145, "delVelocity"=0.0}, {"Time"=35.78000000000145, "delVelocity"=0.0}, {"Time"=35.79000000000145, "delVelocity"=0.0}, {"Time"=35.80000000000145, "delVelocity"=0.0}, {"Time"=35.810000000001445, "delVelocity"=0.0}, {"Time"=35.82000000000144, "delVelocity"=0.0}, {"Time"=35.83000000000144, "delVelocity"=0.0}, {"Time"=35.84000000000144, "delVelocity"=0.0}, {"Time"=35.85000000000144, "delVelocity"=0.0}, {"Time"=35.860000000001435, "delVelocity"=0.0}, {"Time"=35.87000000000143, "delVelocity"=0.0}, {"Time"=35.88000000000143, "delVelocity"=0.0}, {"Time"=35.89000000000143, "delVelocity"=0.0}, {"Time"=35.90000000000143, "delVelocity"=0.0}, {"Time"=35.910000000001425, "delVelocity"=0.0}, {"Time"=35.92000000000142, "delVelocity"=0.0}, {"Time"=35.93000000000142, "delVelocity"=0.0}, {"Time"=35.94000000000142, "delVelocity"=0.0}, {"Time"=35.95000000000142, "delVelocity"=0.0}, {"Time"=35.960000000001415, "delVelocity"=0.0}, {"Time"=35.97000000000141, "delVelocity"=0.0}, {"Time"=35.98000000000141, "delVelocity"=0.0}, {"Time"=35.99000000000141, "delVelocity"=0.0}, {"Time"=36.00000000000141, "delVelocity"=0.0}, {"Time"=36.010000000001405, "delVelocity"=0.0}, {"Time"=36.0200000000014, "delVelocity"=0.0}, {"Time"=36.0300000000014, "delVelocity"=0.0}, {"Time"=36.0400000000014, "delVelocity"=0.0}, {"Time"=36.0500000000014, "delVelocity"=0.0}, {"Time"=36.060000000001395, "delVelocity"=0.0}, {"Time"=36.07000000000139, "delVelocity"=0.0}, {"Time"=36.08000000000139, "delVelocity"=0.0}, {"Time"=36.09000000000139, "delVelocity"=0.0}, {"Time"=36.10000000000139, "delVelocity"=0.0}, {"Time"=36.110000000001385, "delVelocity"=0.0}, {"Time"=36.12000000000138, "delVelocity"=0.0}, {"Time"=36.13000000000138, "delVelocity"=0.0}, {"Time"=36.14000000000138, "delVelocity"=0.0}, {"Time"=36.15000000000138, "delVelocity"=0.0}, {"Time"=36.160000000001375, "delVelocity"=0.0}, {"Time"=36.17000000000137, "delVelocity"=0.0}, {"Time"=36.18000000000137, "delVelocity"=0.0}, {"Time"=36.19000000000137, "delVelocity"=0.0}, {"Time"=36.20000000000137, "delVelocity"=0.0}, {"Time"=36.210000000001365, "delVelocity"=0.0}, {"Time"=36.22000000000136, "delVelocity"=0.0}, {"Time"=36.23000000000136, "delVelocity"=0.0}, {"Time"=36.24000000000136, "delVelocity"=0.0}, {"Time"=36.25000000000136, "delVelocity"=0.0}, {"Time"=36.260000000001355, "delVelocity"=0.0}, {"Time"=36.27000000000135, "delVelocity"=0.0}, {"Time"=36.28000000000135, "delVelocity"=0.0}, {"Time"=36.29000000000135, "delVelocity"=0.0}, {"Time"=36.30000000000135, "delVelocity"=0.0}, {"Time"=36.310000000001345, "delVelocity"=0.0}, {"Time"=36.32000000000134, "delVelocity"=0.0}, {"Time"=36.33000000000134, "delVelocity"=0.0}, {"Time"=36.34000000000134, "delVelocity"=0.0}, {"Time"=36.35000000000134, "delVelocity"=0.0}, {"Time"=36.360000000001335, "delVelocity"=0.0}, {"Time"=36.37000000000133, "delVelocity"=0.0}, {"Time"=36.38000000000133, "delVelocity"=0.0}, {"Time"=36.39000000000133, "delVelocity"=0.0}, {"Time"=36.40000000000133, "delVelocity"=0.0}, {"Time"=36.410000000001325, "delVelocity"=0.0}, {"Time"=36.42000000000132, "delVelocity"=0.0}, {"Time"=36.43000000000132, "delVelocity"=0.0}, {"Time"=36.44000000000132, "delVelocity"=0.0}, {"Time"=36.45000000000132, "delVelocity"=0.0}, {"Time"=36.460000000001315, "delVelocity"=0.0}, {"Time"=36.47000000000131, "delVelocity"=0.0}, {"Time"=36.48000000000131, "delVelocity"=0.0}, {"Time"=36.49000000000131, "delVelocity"=0.0}, {"Time"=36.50000000000131, "delVelocity"=0.0}, {"Time"=36.510000000001305, "delVelocity"=0.0}, {"Time"=36.5200000000013, "delVelocity"=0.0}, {"Time"=36.5300000000013, "delVelocity"=0.0}, {"Time"=36.5400000000013, "delVelocity"=0.0}, {"Time"=36.5500000000013, "delVelocity"=0.0}, {"Time"=36.560000000001295, "delVelocity"=0.0}, {"Time"=36.57000000000129, "delVelocity"=0.0}, {"Time"=36.58000000000129, "delVelocity"=0.0}, {"Time"=36.59000000000129, "delVelocity"=0.0}, {"Time"=36.60000000000129, "delVelocity"=0.0}, {"Time"=36.610000000001286, "delVelocity"=0.0}, {"Time"=36.62000000000128, "delVelocity"=0.0}, {"Time"=36.63000000000128, "delVelocity"=0.0}, {"Time"=36.64000000000128, 
